vi "Hologram64.vi"() -> ()   [LabVIEW 2015]
uses:
  <vilib>/Math Plots/3D Math Plots/3D Surface/3D Surface XCtrl/3D Surface.xctl
  <vilib>/Analysis/2dsp.llb/2D Real FFT.vi
  <vilib>/Math Plots/3D Math Plots/3D Surface/3D Surface Datatype/Public/Plot Helper (Matrix).vi
  <vilib>/gmath/interp.llb/Create Mesh Grid (2D) (x,y arrays).vi
  <vilib>/Math Plots/3D Math Plots/3D Surface/3D Surface Datatype/3D Surface Datatype.lvclass
  <vilib>/gmath/NI_Gmath.lvlib
  <vilib>/Analysis/NI_AALPro.lvlib
panel:
  out "Array 2":dbl[][](array[numeric]) format="%#_1g"
  out "Reference Wave 4":picture
  out "Reference Wave 3":picture
  out "Array":dbl[][](array[numeric])
  out "Reference Wave 2":picture
  out "Reference Wave":picture
  out "Object Wave":picture
  out "Original Image 2":refnum<class "3D Plot Datatype.lvclass">[](xcontrol)
  in  "Path":path
  out "Original Image":refnum<class "3D Plot Datatype.lvclass">[](xcontrol)
  # "Change to real!!!!"
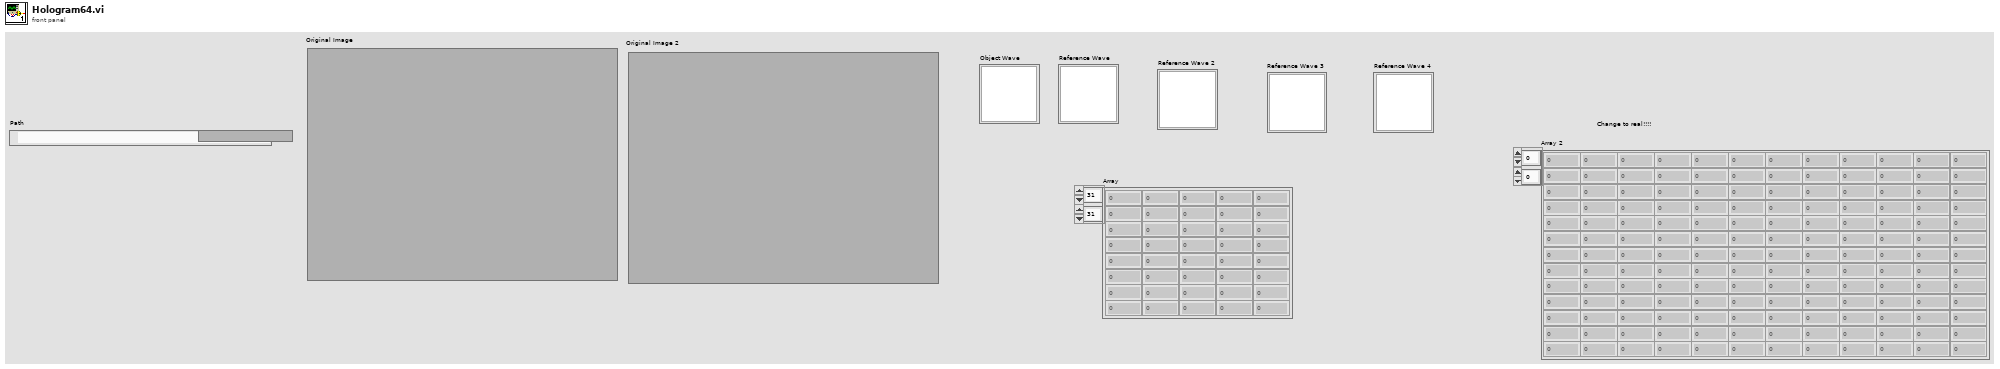
[diagram p1: front panel]
types:
  T1 = typedef "imagedata.ctl" = cluster{"image type":i32, "image depth":i32, "image":u8[], "mask":u8[], "colors":u32[], "Rectangle":cluster{"left":i16, "top":i16, "right":i16, "bottom":i16}}
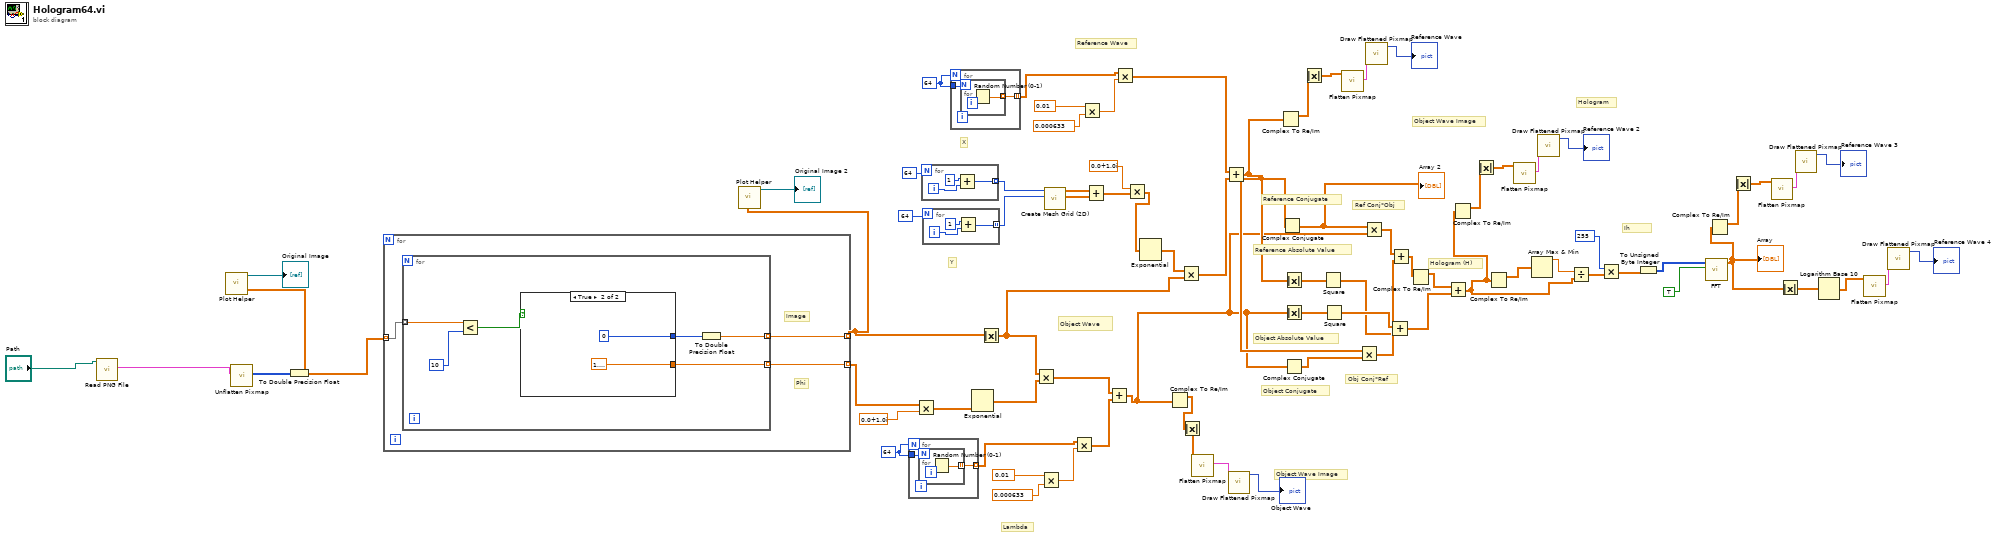
[diagram p0: block diagram]
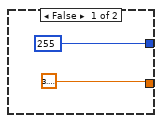
[diagram p2: hidden frame]
diagram:
  w47 = 64
  w68 = 64
  # "Hologram"
  # "Ih"
  # "Hologram (H)"
  # "Ref Conj*Obj"
  # "Obj Conj*Ref"
  # "Reference Conjugate"
  # "Reference Absolute Value"
  # "Object Absolute Value"
  # "Object Conjugate"
  # "Object Wave Image"
  # "Y"
  # "X"
  # "Object Wave Image"
  # "Lambda"
  # "Reference Wave"
  # "Object Wave"
  n1 = call <vilib>:"Read PNG File.vi"("path to PNG file"="Path") -> ("image data"=w75:T1)  [unwired: 8 in, 2 out]
  n2 = call <vilib>:"Unflatten Pixmap.vi"("image data"=w75) -> ("8-bit pixmap"=w78:u8[][])  [unwired: 4 in, 6 out]
  n3 = To Double Precision Float(number=w78) -> (double precision float=w74:dbl[][])
  n4 = call-poly <vilib>:"Plot Helper.vi"("z matrix"=w74) -> ("3D Plot lvclass Array out"=→"Original Image":refnum<class "3D Plot Datatype.lvclass">[])  [unwired: 5 in, 5 out]
  n5 = for {
    tunnel: w74 -> [w81] mode=indexing
    tunnel: [w80] -> w57 mode=indexing
    tunnel: [w79] -> w69 mode=indexing
    # "Phi"
    # "Image"
    n6 = for {
      tunnel: w81 -> [w83] mode=indexing
      tunnel: [w86] -> w80 mode=indexing
      tunnel: [w82] -> w79 mode=indexing
      n7 = Less?(x=w83, y=10) -> (x < y?=w85:bool)
      n8 = case shown="True" w85 {
        tunnel: [255 0] -> w87
        tunnel: [3.141592653589793 1.5707963267948966] -> w82
        frame False {
        }
        frame True {
        }
      }
      n9 = To Double Precision Float(number=w87) -> (double precision float=w86:dbl)
    }
  }
  n10 = call-poly <vilib>:"Plot Helper.vi"("z matrix"=w57) -> ("3D Plot lvclass Array out"=→"Original Image 2":refnum<class "3D Plot Datatype.lvclass">[])  [unwired: 5 in, 5 out]
  n11 = for {
    N: w68 -> [_]
    tunnel: w68 -> [w93]
    tunnel: [w92] -> w65 mode=indexing
    n12 = for {
      N: w93 -> [_]
      tunnel: [w94] -> w92 mode=indexing
      n13 = Random Number (0-1)() -> (number: 0 to 1=w94:dbl)
    }
  }
  n14 = Multiply(x=w69, y=cdb 0.0+1.0i) -> (x*y=w72:cdb[][])
  n15 = for {
    N: 64 -> [_]
    tunnel: [w95] -> w36 mode=indexing
    i -> [w96]
    n16 = Add(x=1, y=w96) -> (x+y=w95:i32)
  }
  n17 = for {
    N: 64 -> [_]
    tunnel: [w98] -> w54 mode=indexing
    i -> [w99]
    n18 = Add(x=1, y=w99) -> (x+y=w98:i32)
  }
  n19 = for {
    N: w47 -> [_]
    tunnel: w47 -> [w102]
    tunnel: [w101] -> w37 mode=indexing
    n20 = for {
      N: w102 -> [_]
      tunnel: [w103] -> w101 mode=indexing
      n21 = Random Number (0-1)() -> (number: 0 to 1=w103:dbl)
    }
  }
  n22 = Exponential(1:w72) -> (0:w71:cdb[][])
  n23 = Absolute Value(x=w57) -> (abs(x)=w52:dbl[][])
  n24 = Multiply(x=w52, y=w71) -> (x*y=w63:cdb[][])
  n25 = Multiply(x=0.01, y=0.000633) -> (x*y=w64:dbl)
  n26 = call-poly <vilib>:"Create Mesh Grid (2D).vi"("y domain"=w54, "x domain"=w36) -> ("Y"=w53:dbl[][], "X"=w35:dbl[][])  [unwired: 7 in, 1 out]
  n27 = Multiply(x=w65, y=w64) -> (x*y=w62:dbl[][])
  n28 = Multiply(x=0.01, y=0.000633) -> (x*y=w44:dbl)
  n29 = Add(x=w35, y=w53) -> (x+y=w50:dbl[][])
  n30 = Add(x=w63, y=w62) -> (x+y=w30:cdb[][])
  n31 = Multiply(x=w37, y=w44) -> (x*y=w43:dbl[][])
  n32 = Multiply(x=cdb 0.0+1.0i, y=w50) -> (x*y=w48:cdb[][])
  n33 = Exponential(1:w48) -> (0:w49:cdb[][])
  n34 = Complex To Re/Im(x + iy=w30) -> (x=w59:dbl[][])  [unwired: 1 out]
  n35 = Multiply(x=w49, y=w52) -> (x*y=w42:cdb[][])
  n36 = Absolute Value(x=w59) -> (abs(x)=w58:dbl[][])
  n37 = call <vilib>:"Flatten Pixmap.vi"("24-bit pixmap"=w58) -> ("image data"=w61:T1)  [unwired: 10 in]
  n38 = Add(x=w43, y=w42) -> (x+y=w32:cdb[][])
  n39 = call <vilib>:"Draw Flattened Pixmap.vi"("image data"=w61) -> ("new picture"=→"Object Wave":picture)  [unwired: 8 in]
  n40 = Complex To Re/Im(x + iy=w32) -> (x=w39:dbl[][])  [unwired: 1 out]
  n41 = Complex Conjugate(1:w32) -> (0:w1:cdb[][])
  "Array 2" <- w1
  n42 = Absolute Value(x=w32) -> (abs(x)=w33:dbl[][])
  n43 = Absolute Value(x=w30) -> (abs(x)=w34:dbl[][])
  n44 = Complex Conjugate(1:w30) -> (0:w31:cdb[][])
  n45 = Absolute Value(x=w39) -> (abs(x)=w38:dbl[][])
  n46 = Square(x=w33) -> (x^2=w26:dbl[][])
  n47 = Square(x=w34) -> (x^2=w29:dbl[][])
  n48 = call <vilib>:"Flatten Pixmap.vi"("24-bit pixmap"=w38) -> ("image data"=w41:T1)  [unwired: 10 in]
  n49 = Multiply(x=w32, y=w31) -> (x*y=w27:cdb[][])
  n50 = Multiply(x=w1, y=w30) -> (x*y=w28:cdb[][])
  n51 = call <vilib>:"Draw Flattened Pixmap.vi"("image data"=w41) -> ("new picture"=→"Reference Wave":picture)  [unwired: 8 in]
  n52 = Add(x=w29, y=w26) -> (x+y=w5:dbl[][])
  n53 = Add(x=w28, y=w27) -> (x+y=w3:cdb[][])
  n54 = Complex To Re/Im(x + iy=w3) -> (x=w2:dbl[][])  [unwired: 1 out]
  n55 = Add(x=w2, y=w5) -> (x+y=w4:dbl[][])
  n56 = Complex To Re/Im(x + iy=w4) -> (x=w20:dbl[][])  [unwired: 1 out]
  n57 = Absolute Value(x=w20) -> (abs(x)=w19:dbl[][])
  n58 = Complex To Re/Im(x + iy=w4) -> (x=w6:dbl[][])  [unwired: 1 out]
  n59 = call <vilib>:"Flatten Pixmap.vi"("24-bit pixmap"=w19) -> ("image data"=w22:T1)  [unwired: 10 in]
  n60 = Array Max & Min(array=w6) -> (max value=w25:dbl)  [unwired: 3 out]
  n61 = call <vilib>:"Draw Flattened Pixmap.vi"("image data"=w22) -> ("new picture"=→"Reference Wave 2":picture)  [unwired: 8 in]
  n62 = Divide(x=w25, y=w4) -> (x/y=w24:dbl[][])
  n63 = Multiply(x=255, y=w24) -> (x*y=w18:dbl[][])
  n64 = To Unsigned Byte Integer(number=w18) -> (unsigned 8bit integer=w17:u8[][])
  n65 = call-poly <vilib>:"FFT.vi"("shift?"=TRUE, "X"=w17) -> ("FFT {X}"=w11:cdb[][])  [unwired: 8 in, 1 out]
  "Array" <- w11
  n66 = Complex To Re/Im(x + iy=w11) -> (x=w13:dbl[][])  [unwired: 1 out]
  n67 = Absolute Value(x=w13) -> (abs(x)=w12:dbl[][])
  n68 = call <vilib>:"Flatten Pixmap.vi"("24-bit pixmap"=w12) -> ("image data"=w15:T1)  [unwired: 10 in]
  n69 = Absolute Value(x=w11) -> (abs(x)=w10:dbl[][])
  n70 = call <vilib>:"Draw Flattened Pixmap.vi"("image data"=w15) -> ("new picture"=→"Reference Wave 3":picture)  [unwired: 8 in]
  n71 = Logarithm Base 10(1:w10) -> (0:w7:dbl[][])
  n72 = call <vilib>:"Flatten Pixmap.vi"("24-bit pixmap"=w7) -> ("image data"=w9:T1)  [unwired: 10 in]
  n73 = call <vilib>:"Draw Flattened Pixmap.vi"("image data"=w9) -> ("new picture"=→"Reference Wave 4":picture)  [unwired: 8 in]
